vi "SR430_interface_ready.vi"(0 "VISA resource name":refnum<visa-resource-name>, 11 "error in (no error)":errorcluster) -> (4 "VISA resource name out":refnum<visa-resource-name>, 8 "interfaceReady?":bool, 15 "error out":errorcluster)   [LabVIEW 2015, in "SR430Driver.lvlib"]
doc: "Checks, if the interface of the instrument is ready (no commands being processed) by querying the standard status byte."
uses:
  SR430Driver.lvlib
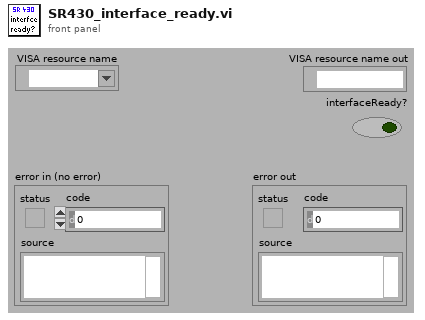
[diagram p1: front panel]
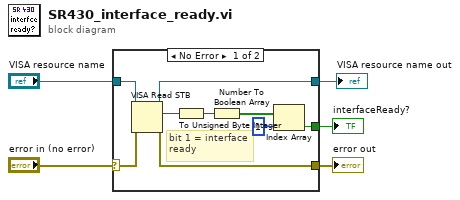
[diagram p0: block diagram]
diagram:
  n1 = case shown="No Error" "error in (no error)" {
    selector: "error in (no error)" -> [w7 w16]
    tunnel: [w14 w16] -> w5
    tunnel: [w13 _] -> w4
    tunnel: "VISA resource name" -> [w8 w15]
    tunnel: [w6 w15] -> w1
    frame No Error {
      # "bit 1 = interface\nready"
      n2 = VISA Read STB(8:w7, 11:w8) -> (0:w14:errorcluster, 2:w10:u16, 3:w6:refnum<visa-resource-name>)
      n3 = To Unsigned Byte Integer(number=w10) -> (unsigned 8bit integer=w9:u8)
      n4 = Number To Boolean Array(number=w9) -> (Boolean array=w11:bool[])
      n5 = Index Array(array=w11, index=1) -> (element=w13:bool)
    }
    frame Error {
    }
  }
  "error out" <- w5
  "interfaceReady?" <- w4
  "VISA resource name out" <- w1
